vi "ESA-C Move Axis To v10.5.2.vi"(0 "Drive Connection Settings":T2={"Objective GPIB-Port"=4, "Stage GPIB-Port"=4, "Drive Selector"=0, "Drive Velocity (V/s)"=5.0} {"Drive Velocity (V/s)" min=10.0 max=160.0 step=0.1 format="%.1f"; "Drive Selector" items=["Obj.", "Stage"]; "Stage GPIB-Port" min=1 max=20 step=1 format="%#.0f"; "Objective GPIB-Port" min=1 max=20 step=1 format="%#.0f"}, 1 "Axis":i32, 2 "Current Voltage (V)":dbl, 3 "Drive New Abs. Positions":T1={"Drive X Set"=10.0, "Drive Y Set"=10.0, "Drive Z Set"=10.0} {"Drive X Set" min=10.0 max=160.0 step=0.1 format="%.1f"; "Drive Z Set" min=10.0 max=160.0 step=0.1 format="%.1f"; "Drive Y Set" min=10.0 max=160.0 step=0.1 format="%.1f"}, 5 "Running":refnum<vi>) -> ()   [LabVIEW 2010]
uses:
  TypeDefs/ESA-C Connection Settings.ctl
  TypeDefs/ESA-C Set Positions.ctl
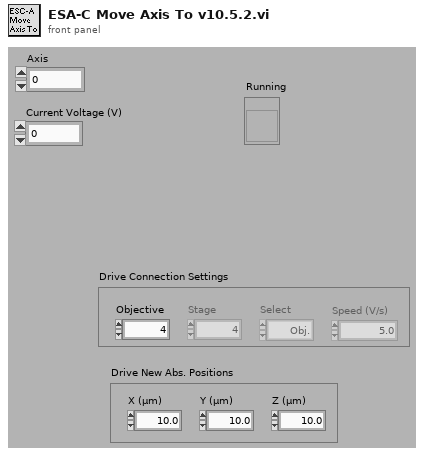
[diagram p1: front panel]
types:
  T1 = typedef "ESA-C Set Positions.ctl" = cluster{"Drive X Set":dbl, "Drive Y Set":dbl, "Drive Z Set":dbl}
  T2 = typedef "ESA-C Connection Settings.ctl" = cluster{"Objective GPIB-Port":i32, "Stage GPIB-Port":i32, "Drive Selector":u16, "Drive Velocity (V/s)":dbl}
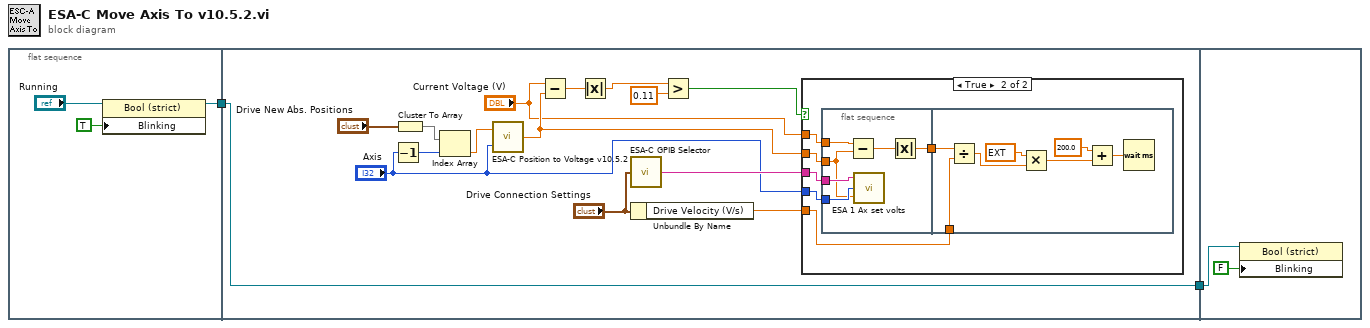
[diagram p0: block diagram]
diagram:
  n1 = flat-sequence {
    tunnel: [w3] -> w1
    tunnel: [w8] -> w2
    tunnel: w1 -> [w8]
    tunnel: w2 -> [w41]
    frame #0 {
      n2 = property class="Bool (strict)"(reference="Running", "Blinking"=TRUE ("Blinkend")) -> (reference out=w3:refnum<vi>)  [unwired: 1 in, 1 out]
    }
    frame #1 {
      n3 = Decrement(x="Axis") -> (x-1=w10:i32)
      n4 = Cluster To Array(cluster="Drive New Abs. Positions") -> (array=w11:dbl[])
      n5 = Index Array(array=w11, index=w10) -> (element=w9:dbl)
      n6 = call "ESA-C Position to Voltage v10.5.2.vi"("Axis"="Axis", "Position (µm)"=w9) -> ("Voltage (V)"=w16:dbl)
      n7 = Subtract(x="Current Voltage (V)", y=w16) -> (x-y=w17:dbl)
      n8 = Absolute Value(x=w17) -> (abs(x)=w18:dbl)
      n9 = call "ESA-C GPIB Selector.vi"("Drive Connection Settings"="Drive Connection Settings") -> ("String"=w14:string)
      n10 = Unbundle By Name("Drive Connection Settings") -> ("Drive Velocity (V/s)"=w6:dbl)
      n11 = Greater?(x=w18, y=0.11) -> (0:w20:bool)
      n12 = case shown="True" w20 {
        tunnel: "Axis" -> [_ w25]
        tunnel: w16 -> [_ w23]
        tunnel: w14 -> [_ w26]
        tunnel: "Current Voltage (V)" -> [_ w24]
        tunnel: w6 -> [_ w21]
        frame False {
        }
        frame True {
          n13 = flat-sequence {
            tunnel: w26 -> [w32]
            tunnel: w25 -> [w31]
            tunnel: w24 -> [w30]
            tunnel: w23 -> [w27]
            tunnel: [w28] -> w22
            tunnel: w22 -> [w39]
            tunnel: w21 -> [w33]
            frame #0 {
              n14 = Subtract(x=w30, y=w27) -> (x-y=w29:dbl)
              n15 = call "ESA 1 Ax set volts.vi"("Voltage"=w27, "Axis"=w31, "GPIB Add"=w32) -> ()
              n16 = Absolute Value(x=w29) -> (abs(x)=w28:dbl)
            }
            frame #1 {
              n17 = Divide(x=w39, y=w33) -> (x/y=w38:dbl)
              n18 = Multiply(x=ext 1000.0, y=w38) -> (x*y=w34:ext)
              n19 = Add(x=200.0, y=w34) -> (x+y=w35:ext)
              n20 = Wait (ms)(milliseconds to wait=w35) -> ()  [unwired: 1 out]
            }
          }
        }
      }
    }
    frame #2 {
      n21 = property class="Bool (strict)"(reference=w41, "Blinking"=FALSE ("Blinkend")) -> ()  [unwired: 1 in, 2 out]
    }
  }
